vi "Get Pointer To Array Copy.vi"(10 "U8 Array":u8[](array[numeric])) -> (2 "Pointer":u32)   [LabVIEW 2021]
panel:
  # "Must dispose of this pointer at some later\npoint to avoid memory leaks."
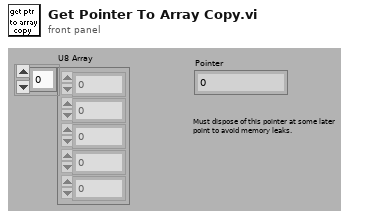
[diagram p1: front panel]
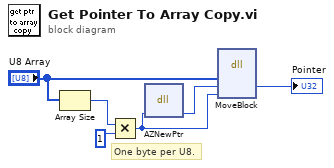
[diagram p0: block diagram]
diagram:
  # "One byte per U8."
  n1 = Array Size(array="U8 Array") -> (size(s)=w2:i32)
  n2 = Multiply(x=w2, y=1) -> (x*y=w1:i32)
  n3 = dll-call lib="LabVIEW" fn="AZNewPtr"("size"=w1) -> (w4:u32)  [unwired: 4 in, 2 out]
  n4 = dll-call lib="LabVIEW" fn="MoveBlock"("src"="U8 Array", "dst"=w4, "size"=w1) -> ("dst"=→"Pointer":u32)  [unwired: 6 in, 2 out]
